vi "set editor class.vi"(8 "error in":errorcluster, 10 "editor class":string, 11 "configuration in":refnum<class "TBM configuration.lvclass">) -> (0 "error out":errorcluster, 3 "configuration out":refnum<class "TBM configuration.lvclass">)   [LabVIEW 2013, in "PL Framework Configuration Tool.lvlib" / "TBM Configuration Node.lvclass"]
uses:
  TBM Configuration Node.lvclass
  <vilib>/NI/Tag Bus Module Framework/root configuration/TBM configuration.lvclass
  <vilib>/NI/CEF/CEF_TreeControl/serializable configuration/NISE_CEF_serializable configuration.lvclass
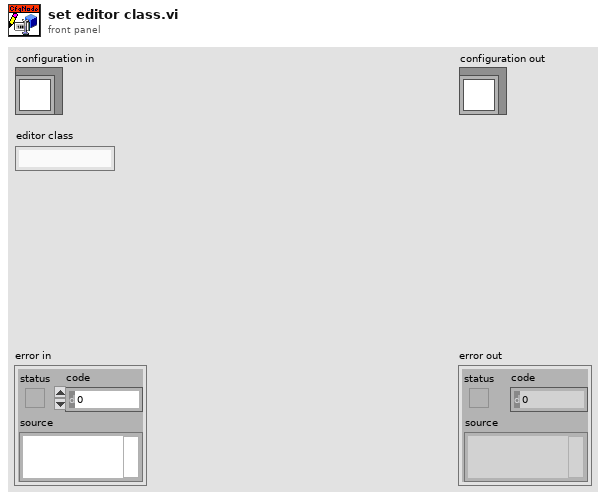
[diagram p1: front panel]
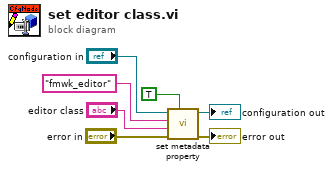
[diagram p0: block diagram]
diagram:
  n1 = call <vilib>:"set metadata property.vi"("overwrite?"=TRUE, "error in"="error in", "value"="editor class", "key"="fmwk_editor", "configuration in"="configuration in") -> ("error out"=→"error out":errorcluster, "configuration out"=→"configuration out":refnum<class "TBM configuration.lvclass">)  [unwired: 5 in]
